vi "FTW-ProjectManager-GetProjectRef.vi"(0 "Project Manager":refnum<class "FTW-ProjectManager.lvclass">, 11 "error in":errorcluster) -> (4 "Project Manager out":refnum<class "FTW-ProjectManager.lvclass">, 6 "Created Project Reference":refnum<vi>, 15 "error out":errorcluster)   [LabVIEW 2012, in "FTW-ProjectManager.lvclass"]
uses:
  FTW-ProjectManager.lvclass
  FTW-ProjectManager.lvclass/FTW-ProjectManager.ctl
panel:
  # "Inputs"
  # "Outputs"
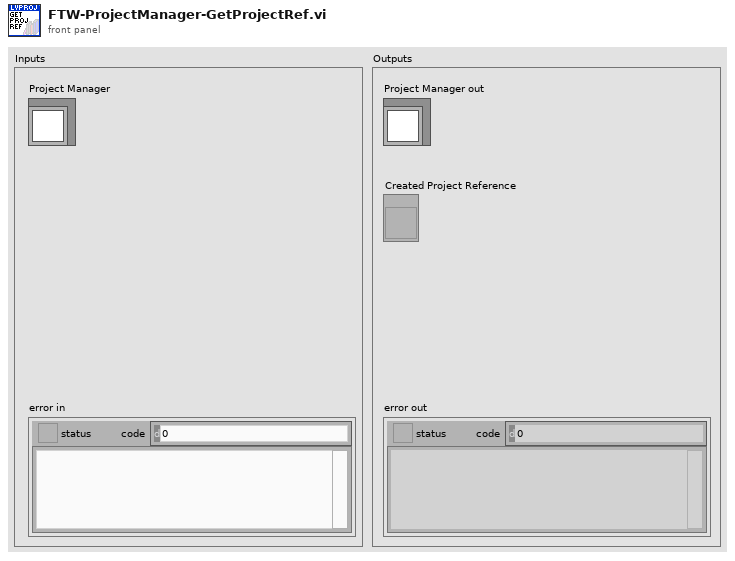
[diagram p1: front panel]
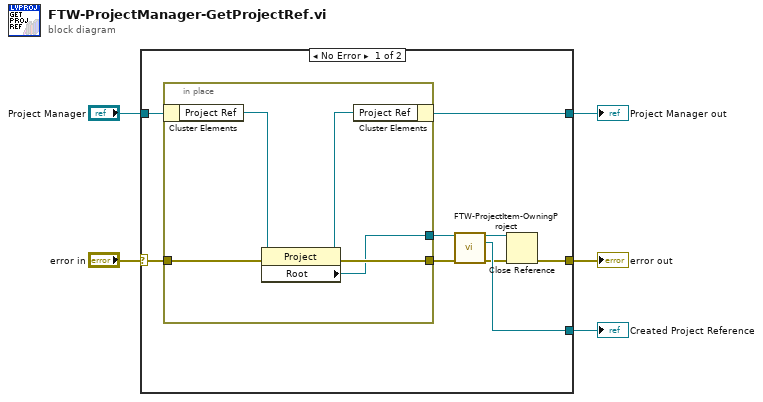
[diagram p0: block diagram]
diagram:
  n1 = case shown="No Error" "error in" {
    selector: "error in" -> [w6 w21]
    tunnel: [w14 w21] -> w5
    tunnel: [w7 w20] -> w3
    tunnel: "Project Manager" -> [w8 w20]
    tunnel: [w12 _] -> w1
    frame No Error {
      n2 = in-place {
        in-place-border: w6 -> [w19]
        in-place-border: [w18] -> w10
        in-place-border: [w17] -> w9
        n3 = in-place-cluster #1(w8) -> ("Project Ref"=w16:refnum<vi>)
        n4 = property class="Project"(reference=w16, error in=w19) -> (reference out=w15:refnum<vi>, error out=w18:errorcluster, "Root"=w17:refnum<vi>)
        n5 = in-place-cluster #1("Project Ref"=w15) -> (w7:refnum<class "FTW-ProjectManager.lvclass">)
      }
      n6 = call "FTW-ProjectItem-OwningProject.vi"("ProjectItem"=w9, "error in"=w10) -> ("ProjectItem out"=w13:refnum<vi>, "Project"=w12:refnum<vi>, "error out"=w11:errorcluster)  [unwired: 11 in]
      n7 = Close Reference(reference=w13, error in (no error)=w11) -> (error out=w14:errorcluster)
    }
    frame Error {
    }
  }
  "error out" <- w5
  "Project Manager out" <- w3
  "Created Project Reference" <- w1
